vi "Esercitazione 3 - Somma4 SubVI on-off.vi"() -> ()   [LabVIEW 2018]
panel:
  out "RISULTATO":dbl
  in  "ON/OFF":bool
  out "STATO":bool
  in  "D":dbl
  in  "C":dbl
  in  "B":dbl
  in  "A":dbl
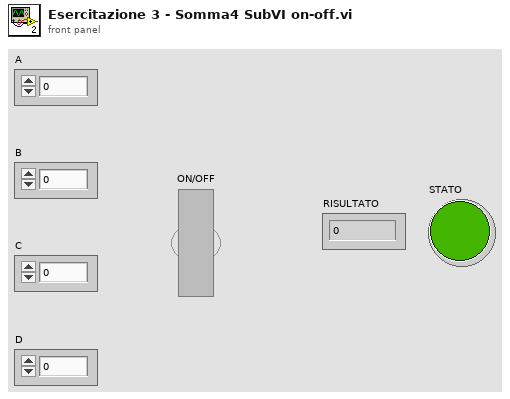
[diagram p1: front panel]
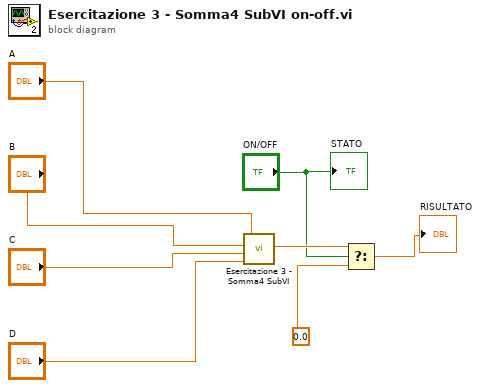
[diagram p0: block diagram]
diagram:
  n1 = call "Esercitazione 3 - Somma4 SubVI.vi"("Numeric Control 4"="D", "Numeric Control 3"="C", "Numeric Control 2"="B", "Numeric Control"="A") -> ("Numeric Indicator"=w2:dbl)
  n2 = Select(t=w2, s="ON/OFF", f=0.0) -> (s? t:f=→"RISULTATO":dbl)
  "STATO" <- "ON/OFF"
